vi "checkAndCreateFile.vi"(2 "filename":string, 3 "path in":path) -> (0 "filename out":string, 1 "path out":path)   [LabVIEW 2021]
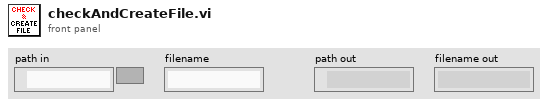
[diagram p1: front panel]
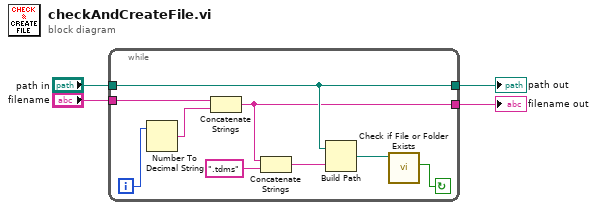
[diagram p0: block diagram]
diagram:
  n1 = while {
    tunnel: "filename" -> [w10]
    tunnel: "path in" -> [w6]
    tunnel: [w6] -> w3
    tunnel: [w5] -> w4
    i -> [w12]
    stop <- w13 continue-if-true
    n2 = Number To Decimal String(number=w12) -> (decimal integer string=w11:string)  [unwired: 1 in]
    n3 = Concatenate Strings(w10, w11) -> (w5:string)
    n4 = Concatenate Strings(w5, ".tdms") -> (w8:string)
    n5 = Build Path(base path=w6, name or relative path=w8) -> (appended path=w7:path)
    n6 = call <vilib>:"Check if File or Folder Exists.vi"("path"=w7) -> ("file or folder exists?"=w13:bool)  [unwired: 1 in, 9 out]
  }
  "filename out" <- w4
  "path out" <- w3
